vi "CryoCooler Alarm Check.vi"(8 "error in (no error)":errorcluster, 10 "Cryo Alarms":T1, 11 "Array":T3[](array[typedef])) -> (0 "error out":errorcluster, 1 "shutdown?":bool, 2 "Alarms":T2[](array[typedef]), 3 "Alarm":bool)   [LabVIEW 2024]
uses:
  Cryo Cooler/CryoCoolerAVC/CryoCoolerAVC Status Cluster.ctl
  typedefs/CC cluster Alarm Data.ctl
  CryoCooler cluster Alarm Settings.ctl
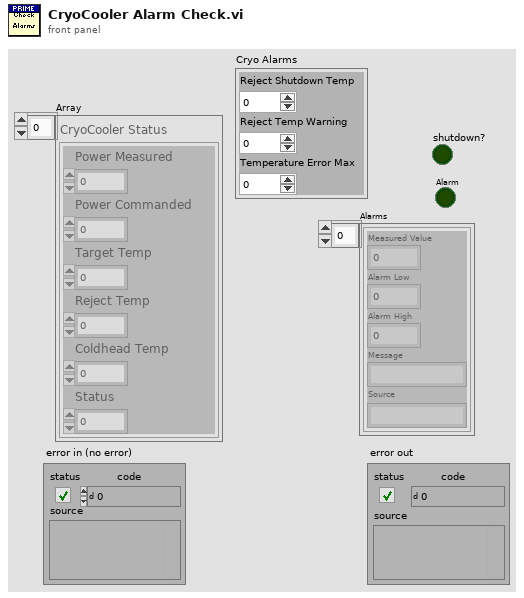
[diagram p1: front panel]
types:
  T1 = typedef "CryoCooler cluster Alarm Settings.ctl" = cluster{"Reject Shutdown Temp":dbl, "Reject Temp Warning":dbl, "Temperature Error Max":dbl}
  T2 = typedef "CC cluster Alarm Data.ctl" = cluster{"Measured Value":dbl, "Alarm Low":dbl, "Alarm High":dbl, "Message":string, "Source":string}
  T3 = typedef "CryoCoolerAVC Status Cluster.ctl" = cluster{"Power Measured":dbl, "Power Commanded":dbl, "Target Temp":dbl, "Reject Temp":dbl, "Coldhead Temp":dbl, "Status":dbl}
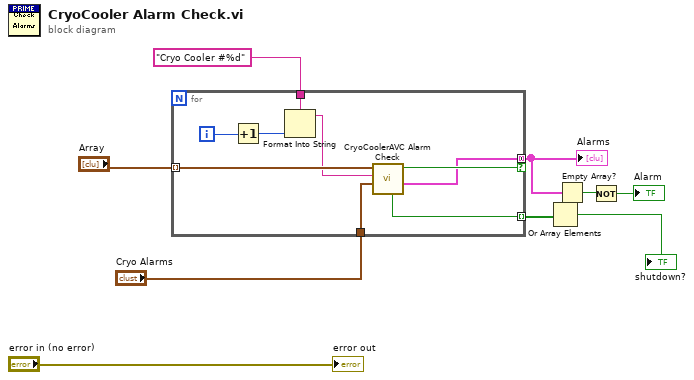
[diagram p0: block diagram]
diagram:
  n1 = for {
    tunnel: "Array" -> [w18] mode=indexing
    tunnel: "Cryo Cooler #%d" ("format string") -> [w17]
    tunnel: [w13] -> w6 mode=concatenating if=w14
    tunnel: "Cryo Alarms" -> [w11]
    tunnel: [w10] -> w2 mode=indexing
    i -> [w16]
    n2 = Increment(x=w16) -> (x+1=w15:i32)
    n3 = Format Into String(format string=w17, w15) -> (resulting string=w12:string)  [unwired: 2 in, 1 out]
    n4 = call "CryoCoolerAVC Alarm Check.vi"("Cryo Alarms"=w11, "Cryocooler"=w12, "CryoCooler Status"=w18) -> ("Alarms"=w13:T2[], "alarm"=w14:bool, "Shutdown?"=w10:bool)  [unwired: 4 in, 2 out]
  }
  "Alarms" <- w6
  n5 = Or Array Elements(Boolean array=w2) -> (logical OR=→"shutdown?":bool)
  n6 = Empty Array?(array=w6) -> (empty?=w5:bool)
  n7 = Not(x=w5) -> (.not. x?=→"Alarm":bool)
  "error out" <- "error in (no error)"
